vi "Connect.vi"(8 "error in (no error)":errorcluster, 11 "PXIe5105 in":refnum<class "PXIe5105.lvclass">) -> (0 "error out":errorcluster, 3 "PXIe5105 out":refnum<class "PXIe5105.lvclass">)   [LabVIEW 2018, in "PXIe5105.lvlib" / "PXIe5105.lvclass"]
doc: "This Override method is used initiative the communication session with the Oscope instrument."
uses:
  PXIe5105.lvclass
  PXIe5105.lvclass/PXIe5105.ctl
  PPLs/Oscilloscope/Parent/Oscilloscope.lvlibp/Oscilloscope.lvclass
  C:/Projects/LabVIEW/PPLs/Oscilloscope/Parent/Oscilloscope.lvlibp/Oscilloscope.lvclass
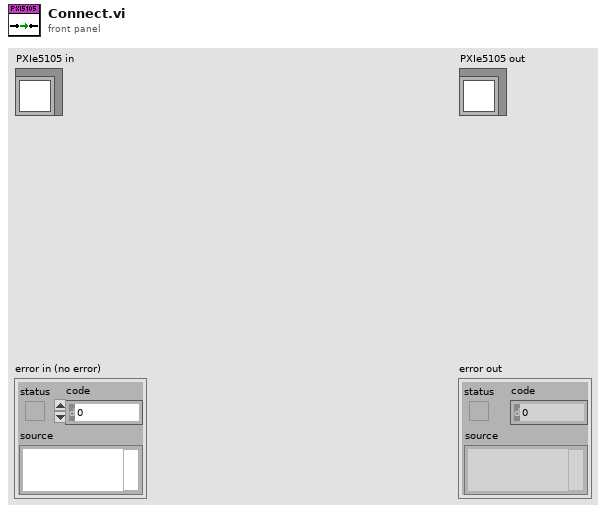
[diagram p1: front panel]
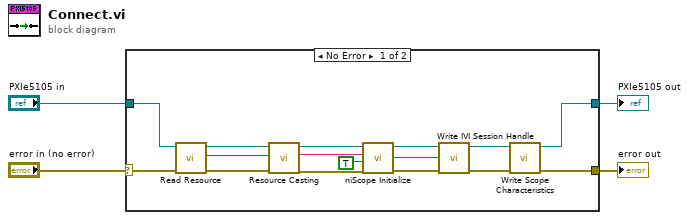
[diagram p0: block diagram]
diagram:
  n1 = case shown="No Error" "error in (no error)" {
    selector: "error in (no error)" -> [w18 w20]
    tunnel: "PXIe5105 in" -> [w19 w21]
    tunnel: [w6 w21] -> w2
    tunnel: [w5 w20] -> w1
    frame No Error {
      n2 = call "Read Resource.vi"("error in (no error)"=w18, "Oscilloscope in"=w19) -> ("error out"=w15:errorcluster, "Resource"=w16:refnum<visa-resource-name>, "Oscilloscope out"=w13:refnum<class "PXIe5105.lvclass">)  [unwired: 7 in]
      n3 = call "Resource Casting.vi"("error in (no error)"=w15, "VISA Resource In"=w16, "PXIe5105 in"=w13) -> ("error out"=w14:errorcluster, "Resource String"=w12:string, "PXIe5105 out"=w11:refnum<class "PXIe5105.lvclass">)  [unwired: 6 in]
      n4 = call <instrlib>:"niScope Initialize.vi"("resource name"=w12, "reset device"=TRUE, "error in"=w14) -> ("instrument handle"=w9:refnum<k15>, "error out"=w10:errorcluster)  [unwired: 11 in]
      n5 = call "Write IVI Session Handle.vi"("error in (no error)"=w10, "IVI Session Handle"=w9, "PXIe5105 in"=w11) -> ("error out"=w7:errorcluster, "PXIe5105 out"=w8:refnum<class "PXIe5105.lvclass">)  [unwired: 7 in]
      n6 = call "Write Scope Characteristics.vi"("error in (no error)"=w7, "PXIe5105 in"=w8) -> ("error out"=w5:errorcluster, "PXIe5105 out"=w6:refnum<class "PXIe5105.lvclass">)  [unwired: 8 in]
    }
    frame Error {
    }
  }
  "error out" <- w1
  "PXIe5105 out" <- w2
